vi "Continuous Waveform Convolution for 1 Chan.vi"(6 "delay output with half kernel length":bool, 7 "reset":bool, 8 "error in (no error)":errorcluster, 9 "algorithm":enum32{"direct", "frequency domain"}(ring)=enum."frequency domain", 10 "kernel":dbl[](array[numeric]), 11 "signal in":waveform(dbl)={"t0"=timestamp(0 s since 1904-01-01), "dt"=0.0, "Y"=[]}) -> (0 "error out":errorcluster, 3 "signal out":waveform(dbl))   [LabVIEW 2020, in "NI_MAPro.lvlib"]
doc: "Convolves single or multiple waveforms and one or more kernels with state, allowing subsequent calls to be processed in a continuous manner. If you are convolving multiple waveforms, the VI maintains separate convolution states for each waveform."
uses:
  NI_MAPro.lvlib
  NI_MABase.lvlib
panel:
  # "Continuous Convolution with Kernel Array"
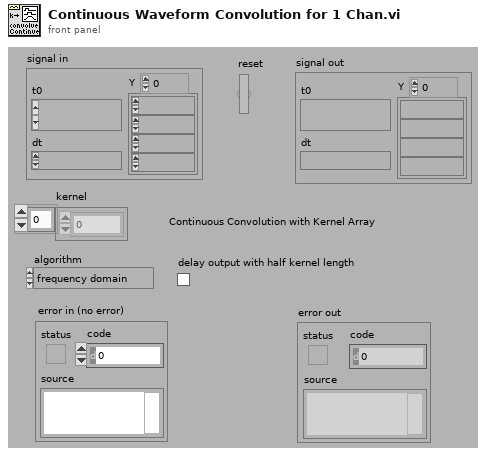
[diagram p1: front panel]
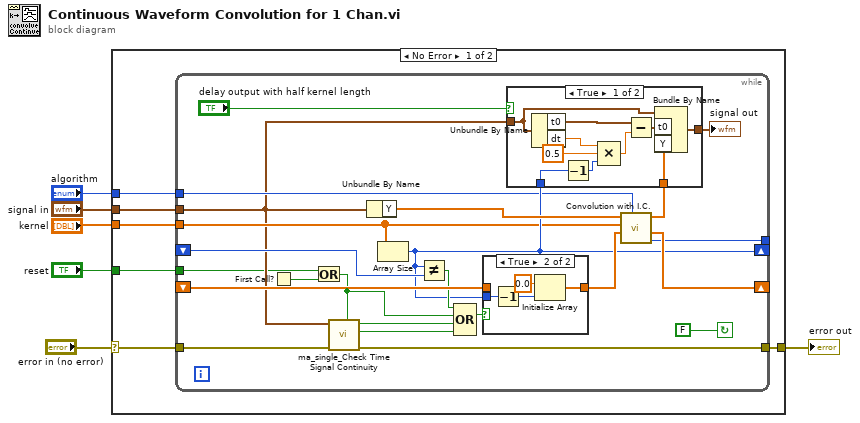
[diagram p0: block diagram]
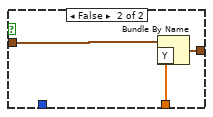
[diagram p2: hidden frame]
diagram:
  n1 = case shown="No Error" "error in (no error)" {
    selector: "error in (no error)" -> [w9 w54]
    tunnel: [w8 w54] -> w5
    tunnel: "algorithm" -> [w12 _]
    tunnel: "signal in" -> [w10 _]
    tunnel: "kernel" -> [w11 _]
    tunnel: "reset" -> [w7 _]
    frame No Error {
      n2 = while {
        shift-right: [w32] -> _
        shift-left: _ -> [w34]
        shift-right: [w23] -> _
        shift-left: _ -> [w31]
        tunnel: [w25] -> _
        tunnel: w12 -> [w22]
        tunnel: w10 -> [w20]
        tunnel: w11 -> [w21]
        tunnel: w9 -> [w19]
        tunnel: [w14] -> w8
        tunnel: w7 -> [w13]
        stop <- FALSE continue-if-true
        n3 = First Call?() -> (First Call?: T/F=w18:bool)
        n4 = Or(x=w13, y=w18) -> (x .or. y?=w15:bool)
        n5 = call "ma_single_Check Time Signal Continuity.vi"("Ignore input time stamp"=w15, "error in (no error)"=w19, "Waveform"=w20) -> ("error out"=w14:errorcluster, "dt changed"=w17:bool, "t0 changed"=w16:bool)  [unwired: 5 in, 1 out]
        n6 = Unbundle By Name(w20) -> ("Y"=w30:dbl[])
        n7 = Array Size(array=w21) -> (size(s)=w23:i32)
        n8 = Not Equal?(x=w23, y=w31) -> (x != y?=w27:bool)
        n9 = Compound Arithmetic op=OR(w27, w15, w16, w17) -> (w26:bool)
        n10 = case shown="True" w26 {
          tunnel: [w49 w53] -> w33
          tunnel: w34 -> [w49 _]
          tunnel: w23 -> [_ w50]
          frame False {
          }
          frame True {
            n11 = Decrement(x=w50) -> (x-1=w51:i32)
            n12 = Initialize Array(0.0 ("element"), w51) -> (w53:dbl[])
          }
        }
        n13 = call "Convolution with I.C..vi"("algorithm"=w22, "Initial conditions"=w33, "Kernel"=w21, "Array in"=w30) -> ("error"=w25:i32, "final conditions"=w32:dbl[], "Array out"=w28:dbl[])  [unwired: 2 in]
        n14 = case shown="True" "delay output with half kernel length" {
          tunnel: [w45 w48] -> w29
          tunnel: w28 -> [w44 w47]
          tunnel: w20 -> [w43 w46]
          tunnel: w23 -> [w39 _]
          frame True {
            n15 = Unbundle By Name(w43) -> ("t0"=w41:timestamp, "dt"=w40:dbl)
            n16 = Decrement(x=w39) -> (x-1=w36:i32)
            n17 = Compound Arithmetic op=MULTIPLY(w40, 0.5, w36) -> (w38:dbl)
            n18 = Subtract(x=w41, y=w38) -> (x-y=w42:timestamp)
            n19 = Bundle By Name(cluster=w43, "t0"=w42, "Y"=w44) -> (w45:waveform(dbl))
          }
          frame False {
            n20 = Bundle By Name(cluster=w46, "Y"=w47) -> (w48:waveform(dbl))
          }
        }
        "signal out" <- w29
      }
    }
    frame Error {
    }
  }
  "error out" <- w5
